vi "LoadSettingsAndCalibration.vi"(8 "error in (no error)":errorcluster, 11 "Cluster in":T1={"Calibration Input"=[], "CalibrationResults"={"Center in Pixels"=[374.0120339529387, 375.46592887074246], "Angle"=0.022945275255000355, "Pixels/MHz X"=0.0, "Pixels/MHz Y"=0.0}, "Highlight"=[], "Running Script"=refnum}) -> (0 "error out":errorcluster, 3 "Cluster out":T1={"Calibration Input"=[], "CalibrationResults"={"Center in Pixels"=[374.0120339529387, 375.46592887074246], "Angle"=0.022945275255000355, "Pixels/MHz X"=0.0, "Pixels/MHz Y"=0.0}, "Highlight"=[], "Running Script"=refnum})   [LabVIEW 2017]
uses:
  TypeDefinitions/ExperimentVariables.ctl
  <vilib>/Utility/xml.llb/Read From XML File(string).vi
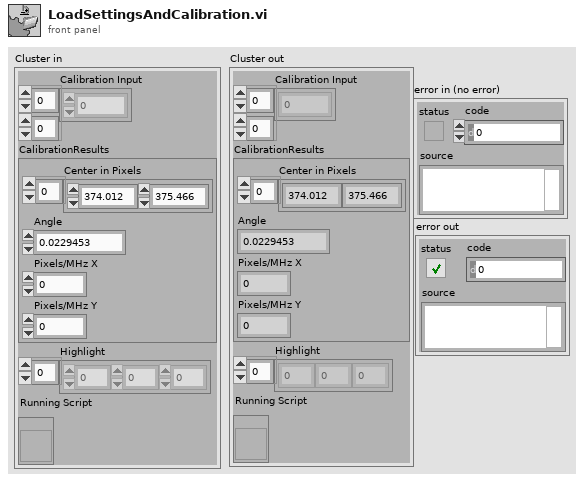
[diagram p1: front panel]
types:
  T1 = typedef "ExperimentVariables.ctl" = cluster{"Calibration Input":i32[][], "CalibrationResults":cluster{"Center in Pixels":dbl[], "Angle":dbl, "Pixels/MHz X":dbl, "Pixels/MHz Y":dbl}, "Highlight":i32[], "Running Script":refnum<vi>}
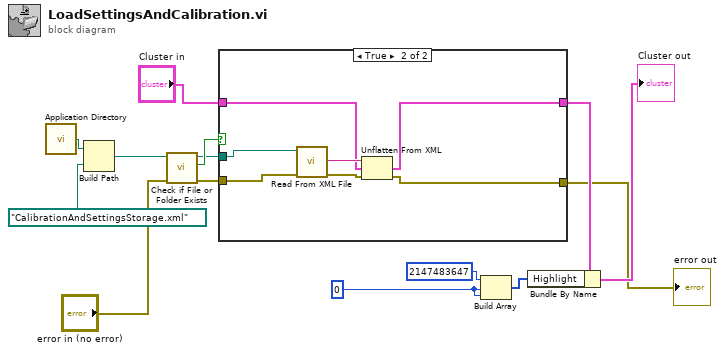
[diagram p0: block diagram]
diagram:
  w5 = 0
  n1 = call <vilib>:"Application Directory.vi"() -> ("Application Directory"=w14:path)
  n2 = Build Path(base path=w14, name or relative path=path "CalibrationAndSettingsStorage.xml" ("XML File Path")) -> (appended path=w12:path)
  n3 = call <vilib>:"Check if File or Folder Exists.vi"("error in (no error)"="error in (no error)", "path"=w12) -> ("error out"=w2:errorcluster, "file or folder exists?"=w11:bool, "dup path"=w10:path)  [unwired: 7 in]
  n4 = case shown="True" w11 {
    tunnel: w10 -> [_ w22]
    tunnel: "Cluster in" -> [w16 w21]
    tunnel: [w16 w20] -> w8
    tunnel: [w15 w17] -> w1
    tunnel: w2 -> [w15 w19]
    frame False {
    }
    frame True {
      n5 = call-poly <vilib>:"Read From XML File.vi"("error in (no error)"=w19, "XML File Path"=w22) -> ("error out"=w18:errorcluster, "XML Elements"=w23:string)  [unwired: 7 in, 1 out]
      n6 = Unflatten From XML(xml string=w23, type=w21, error in (no error)=w18) -> (value=w20:T1, error out=w17:errorcluster)
    }
  }
  "error out" <- w1
  n7 = Build Array(2147483647, w5, w5) -> (w4:i32[])
  n8 = Bundle By Name(cluster=w8, "Highlight"=w4) -> (→"Cluster out":T1)
